vi "智能鞋柜1.vi"() -> ()   [LabVIEW 2018]
panel:
  in  "滑动杆":dbl(slide) scale=0.0..10.0
  out "二维图片":picture
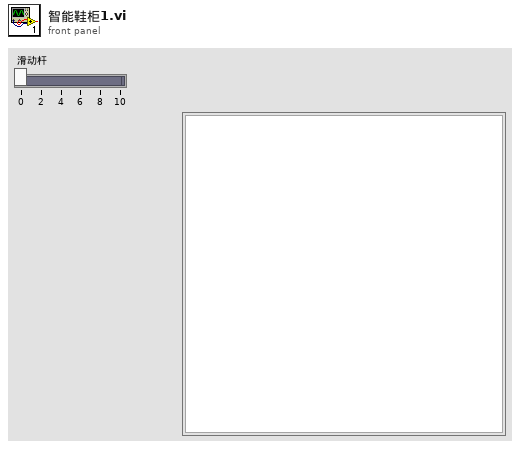
[diagram p1: front panel]
types:
  T1 = typedef "imagedata.ctl" = cluster{"image type":i32, "image depth":i32, "image":u8[], "mask":u8[], "colors":u32[], "Rectangle":cluster{"left":i16, "top":i16, "right":i16, "bottom":i16}}
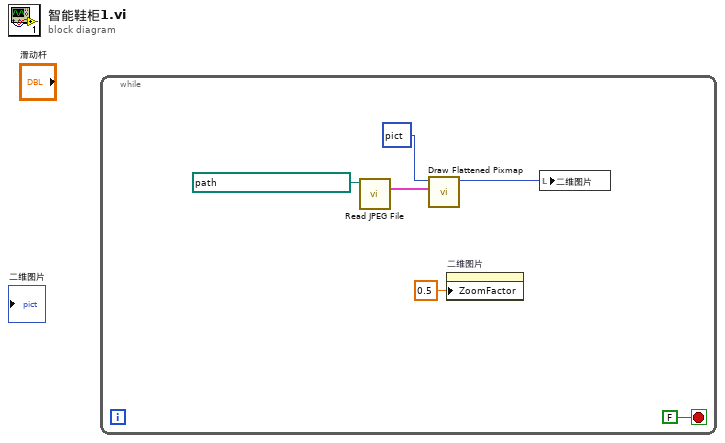
[diagram p0: block diagram]
diagram:
  n1 = while {
    stop <- FALSE stop-if-true
    n2 = call <vilib>:"Read JPEG File.vi"("path to JPEG file"=path "F:/source/图片/18FC.jpeg") -> ("image data"=w5:T1)  [unwired: 8 in, 2 out]
    n3 = call <vilib>:"Draw Flattened Pixmap.vi"("image data"=w5, "picture"=picture data[5B]) -> ("new picture"=w6:picture)  [unwired: 7 in]
    n4 = property on="二维图片" class="Pict"("ZoomFactor"=sgl 0.5 ("缩放因子")) -> ()  [unwired: 2 in, 2 out]
    n5 = local write "二维图片"(w6) -> ()
  }
